vi "set protocols.vi"(8 "error in":errorcluster, 10 "protocol versions":T1, 11 "lvlibretls configurable context in":refnum<class "lvlibretls configurable context.lvclass">) -> (0 "error out":errorcluster, 3 "lvlibretls configurable context out":refnum<class "lvlibretls configurable context.lvclass">)   [LabVIEW 2016, in "lvlibretls configurable context.lvclass"]
uses:
  lvlibretls configurable context.lvclass
  tls protocol versions.ctl
  lvlibretls configurable context.lvclass/lvlibretls configurable context.ctl
  lv tls dll.lvlib
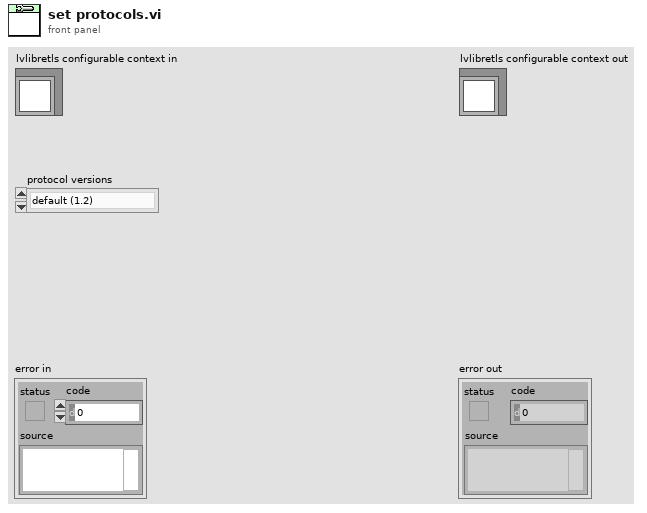
[diagram p1: front panel]
types:
  T1 = typedef "lvlibretls configurable context.lvclass/tls protocol versions.ctl" = enum16{"default (1.2)", "TLS v1.0", "TLS v1.1", "TLS v1.2", "TLS v1.x", "All TLS"}
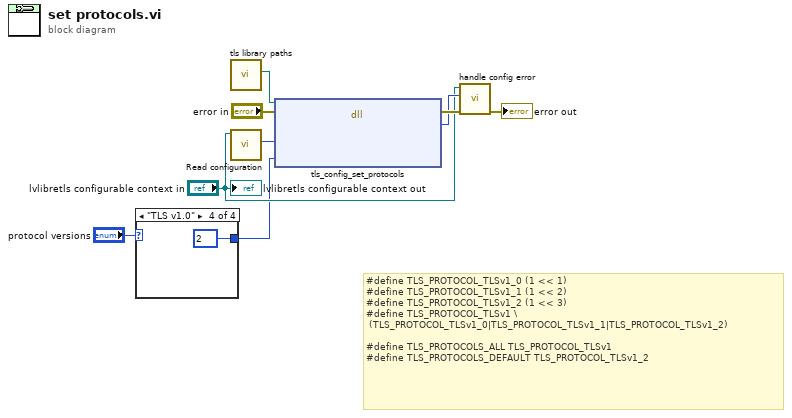
[diagram p0: block diagram]
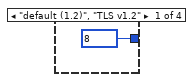
[diagram p2: hidden frame]
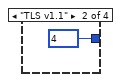
[diagram p3: hidden frame]
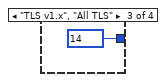
[diagram p4: hidden frame]
diagram:
  # "#define TLS_PROTOCOL_TLSv1_0\t(1 << 1)\n#define TLS_PROTOCOL_TLSv1_1\t(1 << 2)\n#define TLS_PROTOCOL_TLSv1_2\t(1 << 3)\n#define TLS_PROTOCOL_TLSv1 \\\n\t(TLS_PROTOCOL_TLSv1_0|TLS_PROTOCOL_TLSv1_1|TLS_PROTOCOL_TLSv1_2)\n\n#define TLS_PROTOCOLS_ALL TLS_PROTOCOL_TLSv1\n#define TLS_PROTOCOLS_DEFAULT TLS_PROTOCOL_TLSv1_2"
  n1 = case shown="\"TLS v1.0\"" "protocol versions" {
    tunnel: [8 4 14 2] -> w1
    frame "default (1.2)", "TLS v1.2" {
    }
    frame "TLS v1.1" {
    }
    frame "TLS v1.x", "All TLS" {
    }
    frame "TLS v1.0" {
    }
  }
  n2 = call "tls library paths.vi"() -> ("libtls"=w9:path)  [unwired: 8 in, 3 out]
  n3 = call "Read configuration.vi"("lvlibretls configurable context in"="lvlibretls configurable context in") -> ("configuration"=w8:u64)  [unwired: 10 in]
  n4 = dll-call lib="C:/Users/IEUser/Desktop/tlssimple/libtls-15.dll" fn="tls_config_set_protocols"(path in=w9, error in="error in", "config"=w8, "protocol bitset"=w1) -> (error out=w7:errorcluster, "return"=w6:i32)  [unwired: 3 in, 1 out]
  n5 = call "handle config error.vi"("error in"=w7, "return"=w6, "lvlibretls configurable context in"="lvlibretls configurable context in") -> ("error out"=→"error out":errorcluster)  [unwired: 8 in]
  "lvlibretls configurable context out" <- "lvlibretls configurable context in"
